vi "Change Data Type.vi"(8 "error in (no error)":errorcluster, 10 "Data Type Selector Return":string, 11 "DataGrid Config Dialog in":refnum<class "DataGrid Config Dialog.lvclass">) -> (0 "error out":errorcluster, 3 "DataGrid Config Dialog out":refnum<class "DataGrid Config Dialog.lvclass">)   [LabVIEW 2018, in "DataGrid Config Dialog.lvclass"]
uses:
  DataGrid Config Dialog.lvclass
  DataGrid Config Dialog.lvclass/DataGrid Config Dialog.ctl
  Data Type Classes/Generic/Generic Data Type.lvclass/Generic Data Type.ctl
  Data Type Classes/Generic/Write Column Index.vi
  Data Type Classes/Generic/Generic Data Type.lvclass
  DataGrid Config/DataGrid Config.lvclass
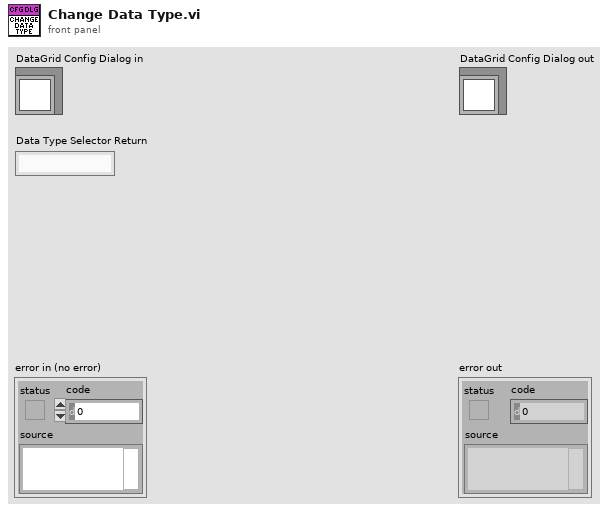
[diagram p1: front panel]
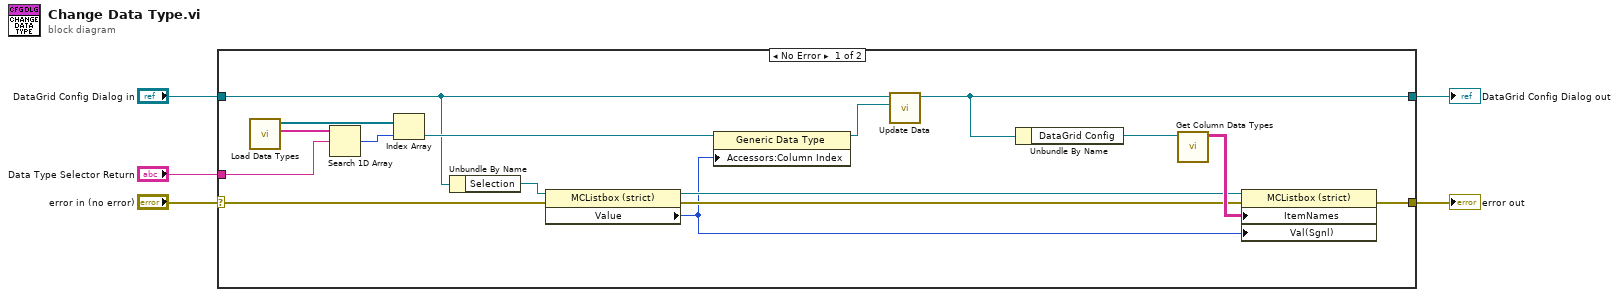
[diagram p0: block diagram]
diagram:
  n1 = case shown="No Error" "error in (no error)" {
    selector: "error in (no error)" -> [w7 w23]
    tunnel: [w17 w23] -> w1
    tunnel: [w10 w22] -> w2
    tunnel: "DataGrid Config Dialog in" -> [w8 w22]
    tunnel: "Data Type Selector Return" -> [w18 _]
    frame No Error {
      n2 = call "Load Data Types.vi"() -> ("Data Type Names"=w21:string[], "Data Type Objects"=w20:refnum<class "Generic Data Type.lvclass">[])  [unwired: 9 in, 1 out]
      n3 = Search 1D Array(1D array=w21, element=w18) -> (index of element=w19:i32)  [unwired: 1 in]
      n4 = Index Array(array=w20, index=w19) -> (element=w16:refnum<class "Generic Data Type.lvclass">)
      n5 = Unbundle By Name(w8) -> ("Selection"=w12:refnum<vi>)
      n6 = property class="MCListbox (strict)"(reference=w12, error in=w7) -> (reference out=w14:refnum<vi>, error out=w13:errorcluster, "Value"=w6:i32)
      n7 = property class="Generic Data Type"(reference=w16, "Accessors:Column Index"=w6) -> (reference out=w11:refnum<class "Generic Data Type.lvclass">)  [unwired: 1 in, 1 out]
      n8 = call "Update Data.vi"("Generic Data Type"=w11, "DataGrid Config Dialog in"=w8) -> ("DataGrid Config Dialog out"=w10:refnum<class "DataGrid Config Dialog.lvclass">)  [unwired: 8 in, 1 out]
      n9 = Unbundle By Name(w10) -> ("DataGrid Config"=w9:refnum<class "DataGrid Config.lvclass">)
      n10 = call "Get Column Data Types.vi"("DataGrid Config"=w9) -> ("Column Data Type Names"=w15:string[][])  [unwired: 10 in]
      n11 = property class="MCListbox (strict)"(reference=w14, error in=w13, "ItemNames"=w15, "Val(Sgnl)"=w6) -> (error out=w17:errorcluster)  [unwired: 1 out]
    }
    frame Error {
    }
  }
  "error out" <- w1
  "DataGrid Config Dialog out" <- w2
